vi "Delete Series.vi"(0 "InfluxDB in":refnum<class "InfluxDB Client.lvclass">, 5 "Database name":string, 7 "Series name":string, 11 "error in (no error)":errorcluster) -> (4 "InfluxDB out":refnum<class "InfluxDB Client.lvclass">, 15 "error out":errorcluster)   [LabVIEW 2017]
doc: "Deletes a time series from a specific database."
uses:
  <vilib>/httpClient/LabVIEWHTTPClient.lvlib
  InfluxDB Client.lvclass
panel:
  out "Status":string
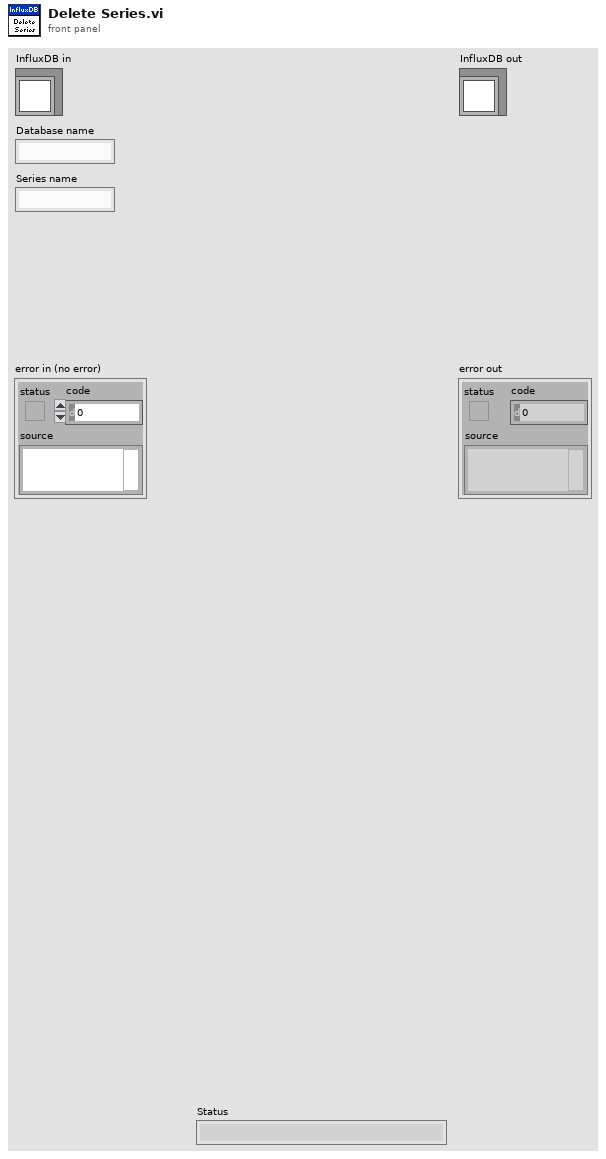
[diagram p1: front panel]
types:
  T1 = typedef "LabVIEWHTTPClient.lvlib/ClientHandle.ctl" = refnum<k1>
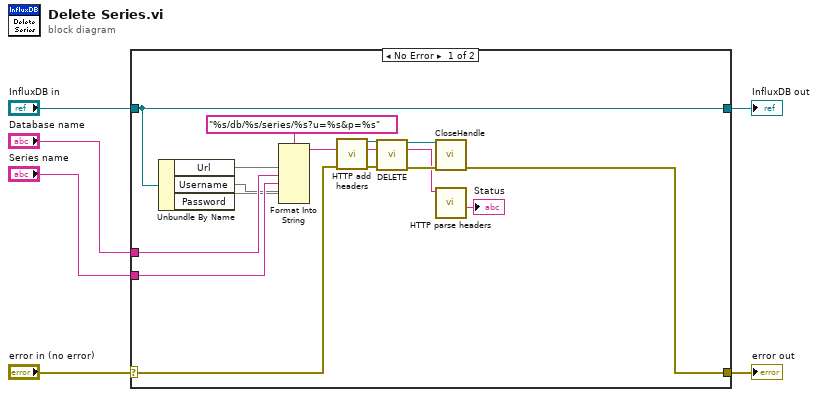
[diagram p0: block diagram]
diagram:
  n1 = case shown="No Error" "error in (no error)" {
    selector: "error in (no error)" -> [w9 w24]
    tunnel: [w16 w24] -> w5
    tunnel: [w22 w23] -> w3
    tunnel: "InfluxDB in" -> [w22 w23]
    tunnel: "Database name" -> [w13 _]
    tunnel: "Series name" -> [w12 _]
    frame No Error {
      n2 = Unbundle By Name(w22) -> ("Url"=w20, "Username"=w11, "Password"=w10)
      n3 = Format Into String(format string="%s/db/%s/series/%s?u=%s&p=%s" ("url"), w20, w13, w12, w11, w10) -> (resulting string=w17:string)  [unwired: 2 in, 1 out]
      n4 = call "HTTP add headers.vi"("error in (no error)"=w9) -> ("client handle out"=w7:T1, "error out"=w8:errorcluster)  [unwired: 13 in]
      n5 = call <vilib>:"DELETE.vi"("client handle"=w7, "url"=w17, "error in (no error)"=w8) -> ("client handle out"=w19:T1, "headers"=w15:string, "error out"=w18:errorcluster)  [unwired: 9 in, 1 out]
      n6 = call <vilib>:"CloseHandle.vi"("client handle"=w19, "error in (no error)"=w18) -> ("error out"=w16:errorcluster)  [unwired: 13 in]
      n7 = call "HTTP parse headers.vi"("HTTP headers"=w15) -> ("Status"=→"Status":string)  [unwired: 8 in, 2 out]
    }
    frame Error {
    }
  }
  "error out" <- w5
  "InfluxDB out" <- w3
